vi "Destroy.vi"(0 "reference in":refnum<class "Vision.lvclass">, 5 "error in (no error)":errorcluster) -> (14 "reference out":refnum<class "Vision.lvclass">, 19 "error out":errorcluster)   [LabVIEW 2018, in "Vision.lvclass"]
uses:
  Vision.lvclass
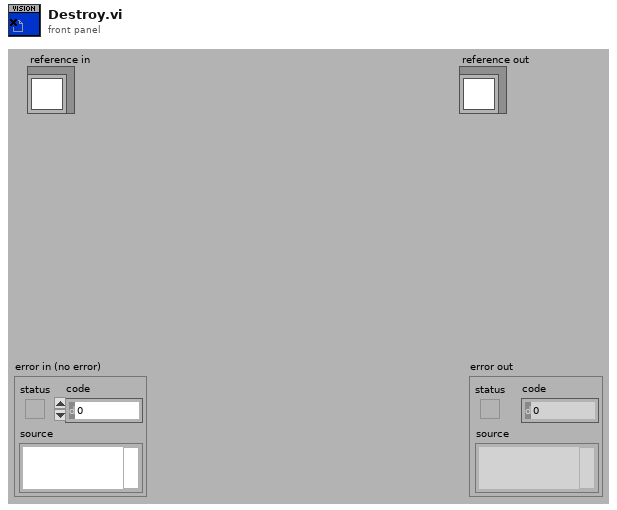
[diagram p1: front panel]
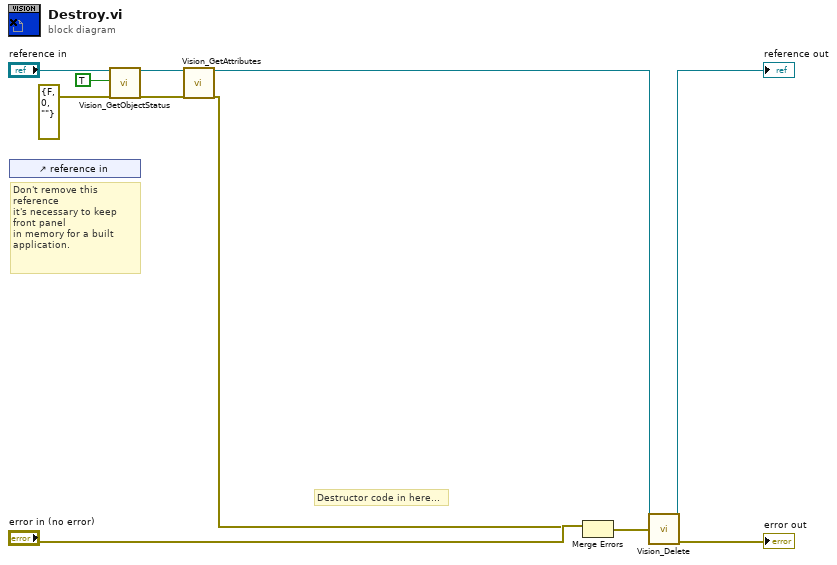
[diagram p0: block diagram]
diagram:
  # "Don't remove this reference\nit's necessary to keep front panel\nin memory for a built application."
  # "Destructor code in here..."
  n1 = control-ref of="reference in"() -> ()  [unwired: 1 out]
  n2 = call "Vision_GetObjectStatus.vi"("reference in"="reference in", "Simple Info"=TRUE, "error in (no error)"=errorcluster {"status"=FALSE, "code"=0, "source"=""}) -> ("reference out"=w5:refnum<class "Vision.lvclass">, "error out"=w2:errorcluster)  [unwired: 6 in, 9 out]
  n3 = call "Vision_GetAttributes.vi"("reference in"=w5, "error in (no error)"=w2) -> ("reference out"=w9:refnum<class "Vision.lvclass">, "error out"=w7:errorcluster)  [unwired: 14 in, 2 out]
  n4 = Merge Errors("error in (no error)", w7) -> (w8:errorcluster)
  n5 = call "Vision_Delete.vi"("reference in"=w9, "error in (no error)"=w8) -> ("reference out"=→"reference out":refnum<class "Vision.lvclass">, "error out"=→"error out":errorcluster)  [unwired: 15 in, 1 out]
